vi "GetType.vi"(8 "error in (no error)":errorcluster, 11 "Read Single-Point Msg":refnum<class "Read Single-Point Msg.lvclass">) -> (0 "error out":errorcluster, 2 "Data Sample":variant, 3 "Read Single-Point Msg":refnum<class "Read Single-Point Msg.lvclass">)   [LabVIEW 2016, in "CS++DMM.lvlib" / "Read Single-Point Msg.lvclass"]
uses:
  Read Single-Point Msg.lvclass
  Read Single-Point Msg.lvclass/Read Single-Point Msg.ctl
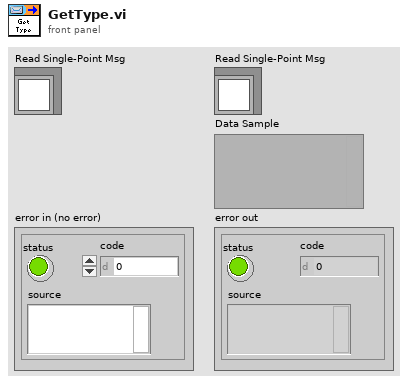
[diagram p1: front panel]
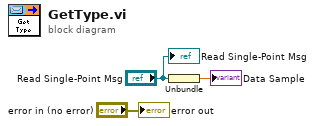
[diagram p0: block diagram]
diagram:
  n1 = Unbundle("Read Single-Point Msg") -> (→"Data Sample":dbl[unit])
  "error out" <- "error in (no error)"
  "Read Single-Point Msg" <- "Read Single-Point Msg"
